vi "Response from Arduino_MI.vi"(8 "error in (no error)":errorcluster, 10 "Message from Arduino":string, 11 "Controls[]":refnum<vi>[](array[refnum])) -> (0 "error out":errorcluster, 2 "Opcode Present":bool, 3 "Index":i32)   [LabVIEW 2019, in "Machine Interface.lvclass"]
uses:
  Machine Interface.lvclass
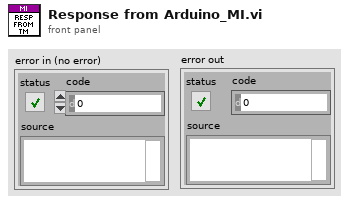
[diagram p1: front panel]
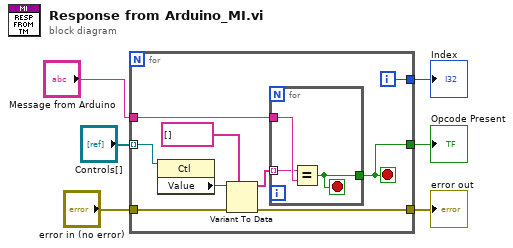
[diagram p0: block diagram]
diagram:
  n1 = for {
    tunnel: "Message from Arduino" -> [w15]
    tunnel: [w14] -> w3
    tunnel: [w10] -> w2
    tunnel: "error in (no error)" -> [w9]
    tunnel: "Controls[]" -> [w8] mode=indexing
    tunnel: [w7] -> w1
    i -> [w14]
    stop <- w7 stop-if-true
    n2 = property class="Ctl"(reference=w8) -> ("Value"=w13:variant)  [unwired: 1 in, 2 out]
    n3 = Variant To Data(error in=w9, type=string[] [], Variant=w13) -> (data=w11:string[], error out=w10:errorcluster)
    n4 = for {
      tunnel: w15 -> [w18]
      tunnel: [w17] -> w7
      tunnel: w11 -> [w16] mode=indexing
      stop <- w17 stop-if-true
      n5 = Equal?(x=w16, y=w18) -> (x = y?=w17:bool)
    }
  }
  "Index" <- w3
  "error out" <- w2
  "Opcode Present" <- w1
